vi "JKI without event handle.vi"(8 "error in":errorcluster, 10 "测试参数":string[](array[string]), 11 "测试命令":string[](array[string])) -> (0 "error out":errorcluster, 3 "执行程序":string)   [LabVIEW 2017]
doc: "函数名称： \n函数功能：无事件结构 JKI状态机模板\n入口参数：\n出口参数：\n创建时间：2018-8-17 编辑者 ：翁赟"
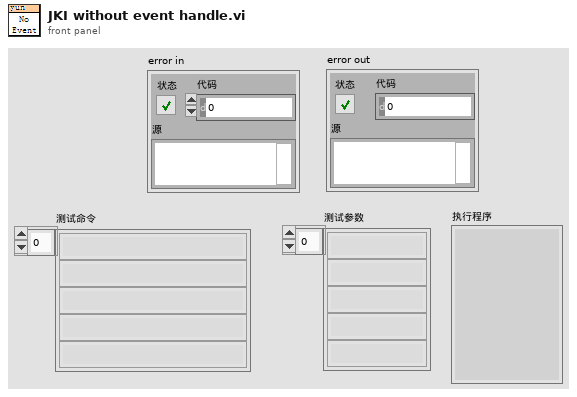
[diagram p1: front panel]
types:
  T1 = enum32{"invalid app kind", "Development System", "Run Time System", "Student Edition", "Embedded LabVIEW", "Evaluation", "Custom"}
  T2 = enum32{"Invalid", "Standard", "Closed", "Hidden", "Minimized", "Maximized"}
  T3 = cluster{"Core":cluster{"Current VI Reference":refnum<vi>, "Close Panel on Exit?":bool}, "Your Boolean data":bool, "Your string data":string}
  T4 = cluster{"Current VI Reference":refnum<vi>, "Close Panel on Exit?":bool}
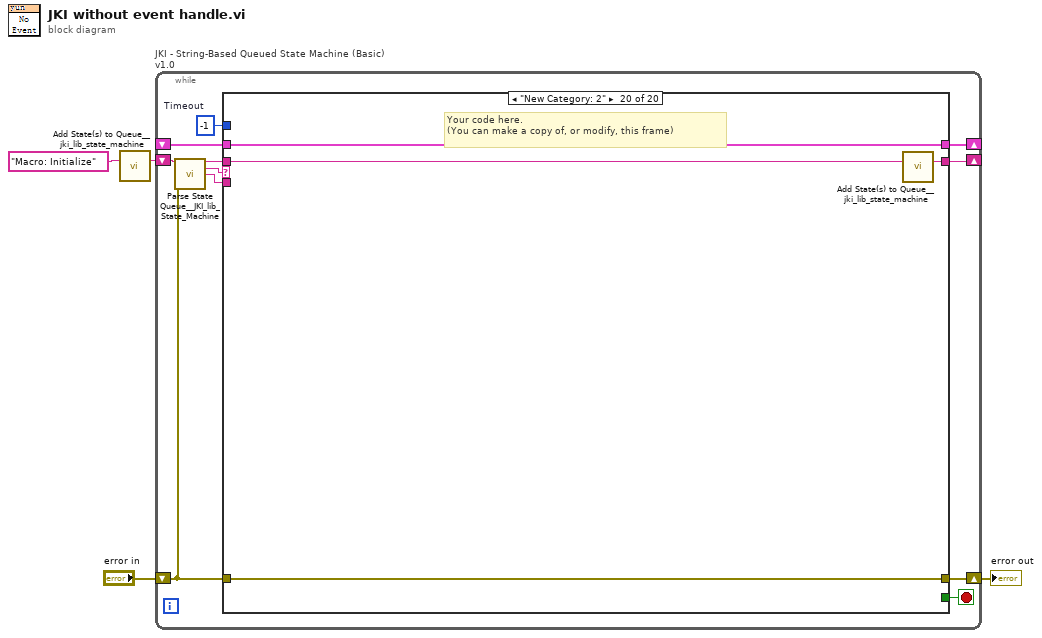
[diagram p0: block diagram]
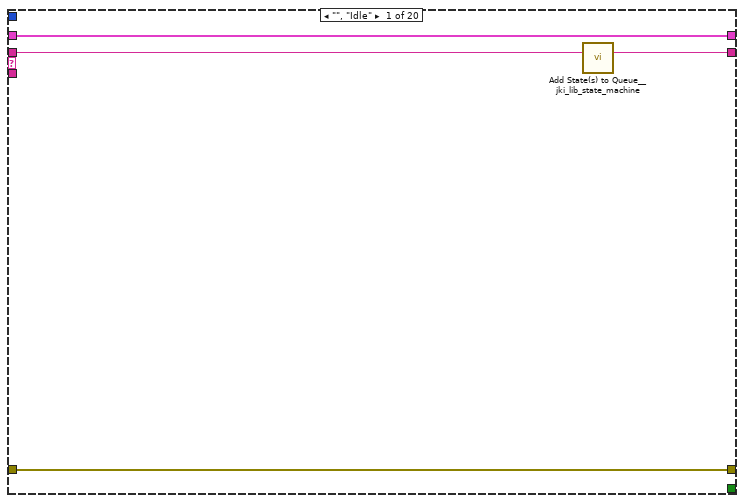
[diagram p2: hidden frame]
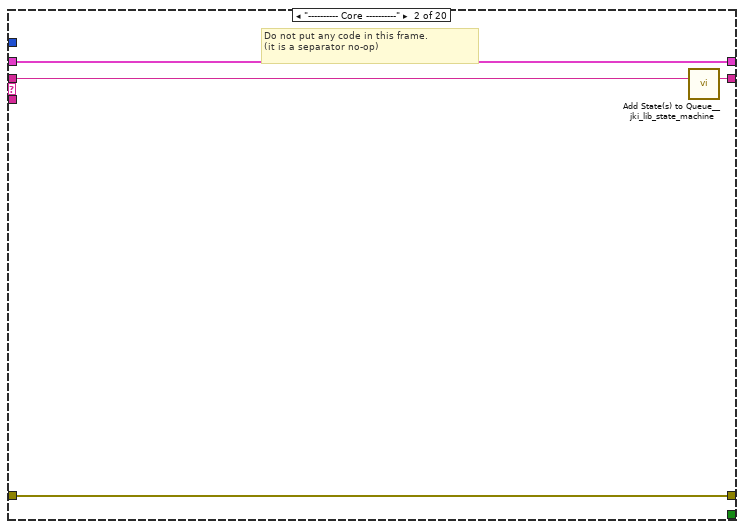
[diagram p3: hidden frame]
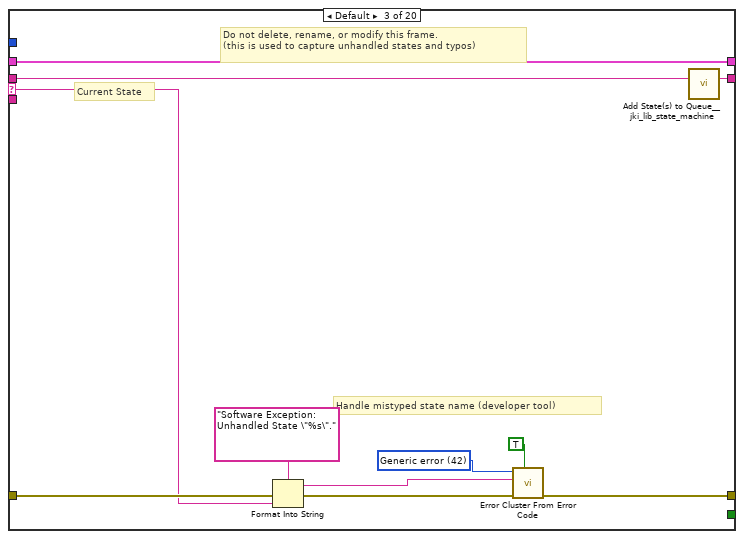
[diagram p4: hidden frame]
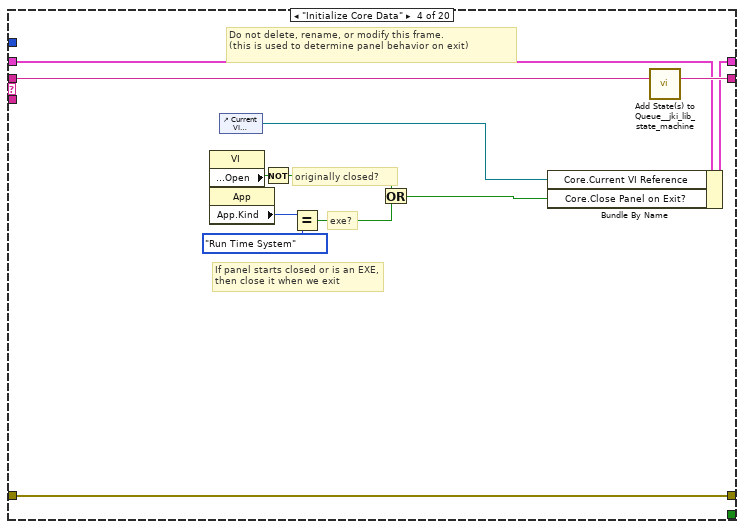
[diagram p5: hidden frame]
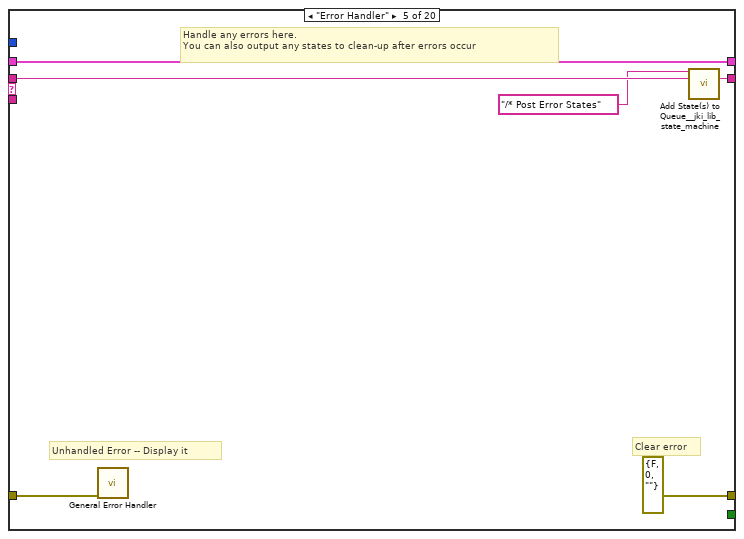
[diagram p6: hidden frame]
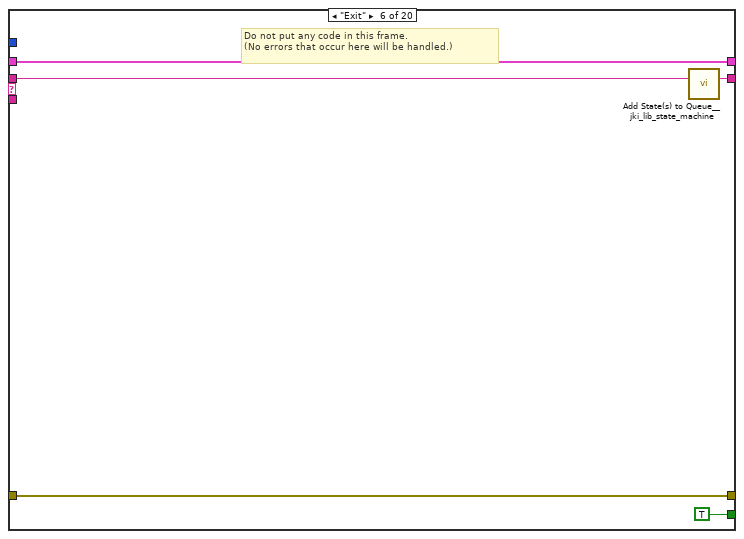
[diagram p7: hidden frame]
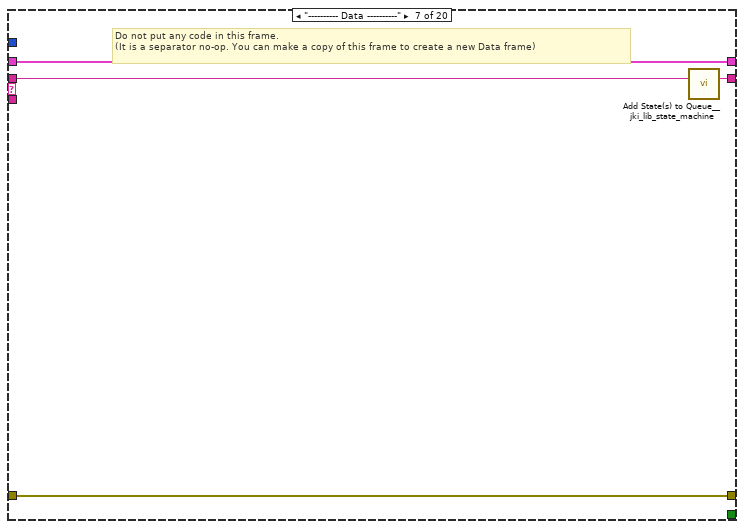
[diagram p8: hidden frame]
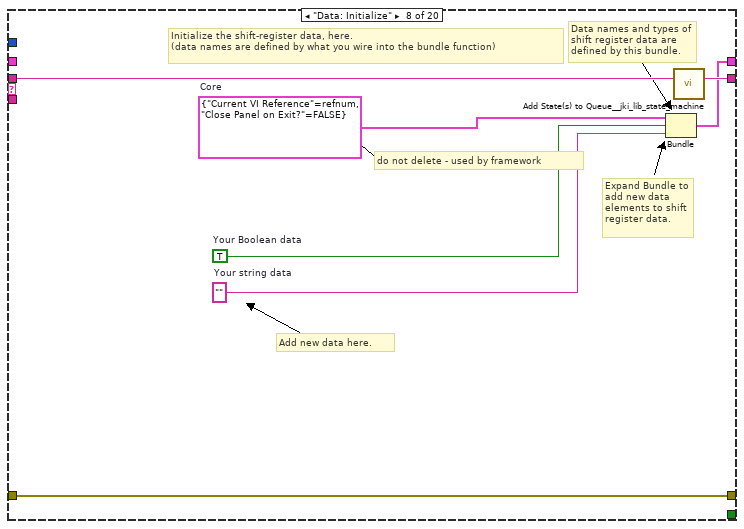
[diagram p9: hidden frame]
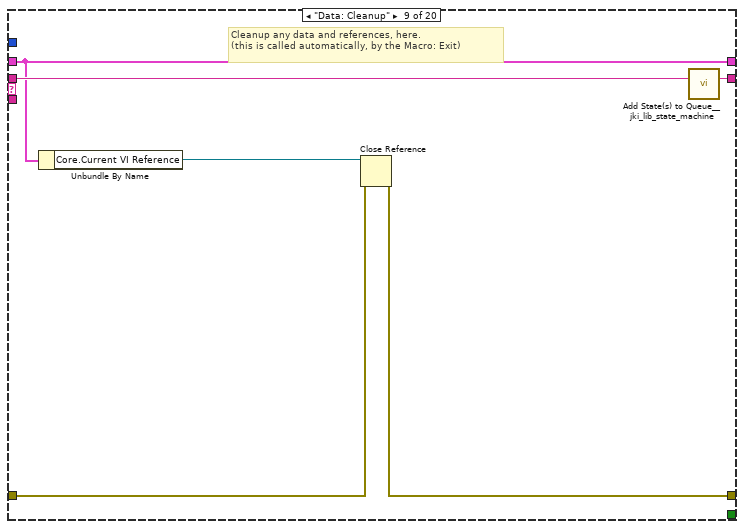
[diagram p10: hidden frame]
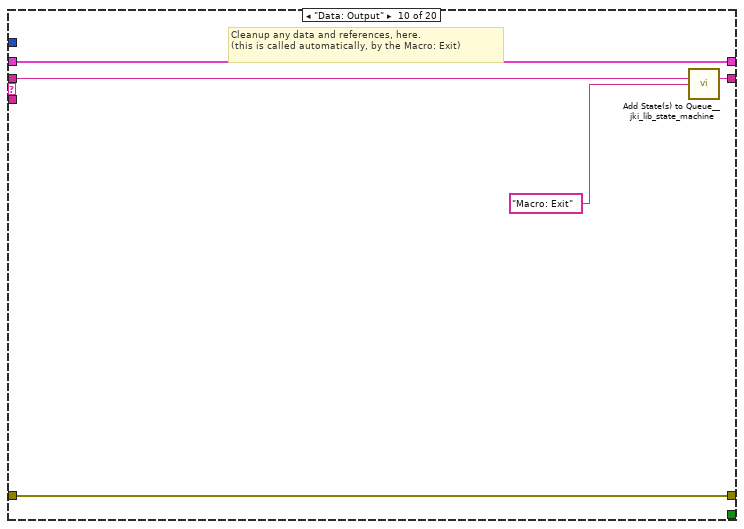
[diagram p11: hidden frame]
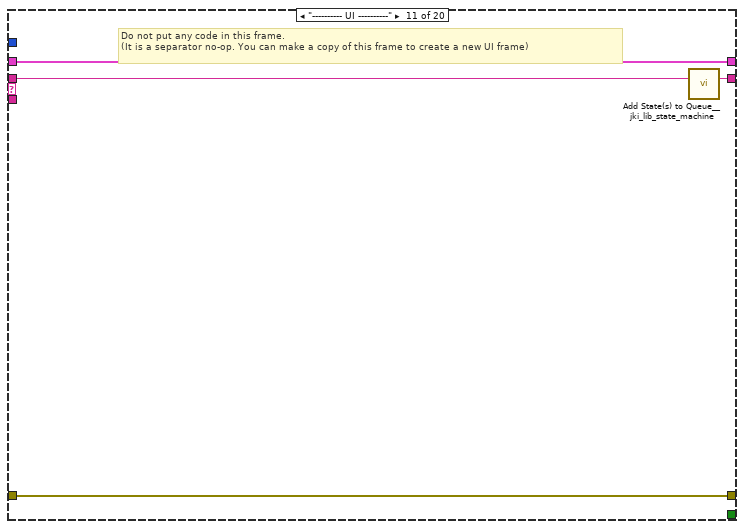
[diagram p12: hidden frame]
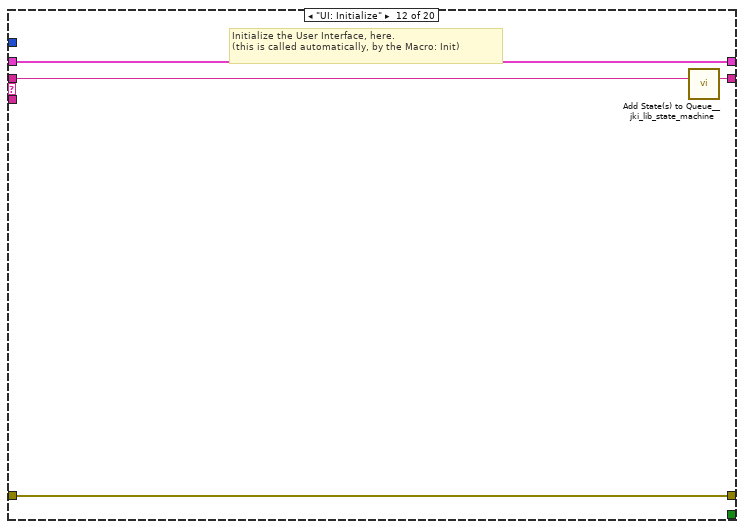
[diagram p13: hidden frame]
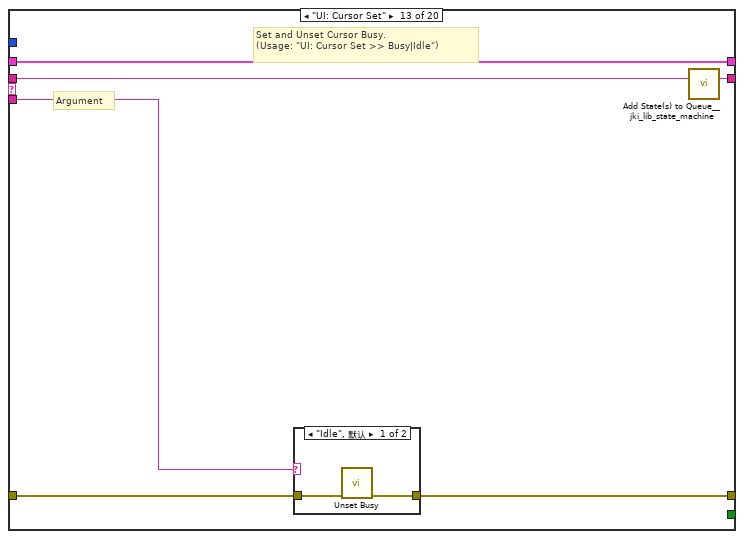
[diagram p14: hidden frame]
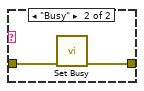
[diagram p15: hidden frame]
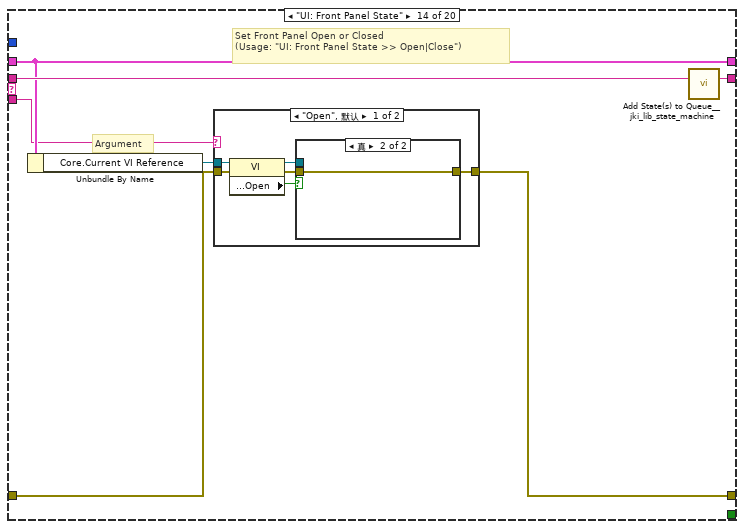
[diagram p16: hidden frame]
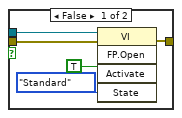
[diagram p17: hidden frame]
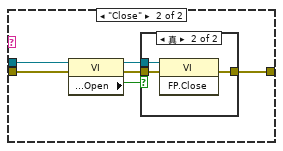
[diagram p18: hidden frame]
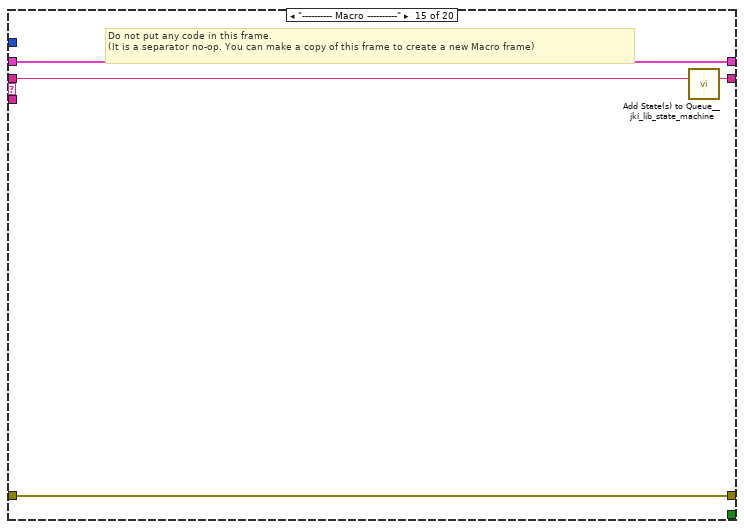
[diagram p20: hidden frame]
diagram:
  n1 = call "Add State(s) to Queue__jki_lib_state_machine.vi"("State(s) in (\"\")"="Macro: Initialize") -> ("States Out"=w4:string)  [unwired: 14 in]
  n2 = while "JKI - String-Based Queued State Machine (Basic) v1.0" {
    shift-right: [w8] -> _
    shift-left: _ -> [w7]
    shift-right: [w11] -> w1
    shift-left: "error in" -> [w5]
    shift-right: [w10] -> _
    shift-left: w4 -> [w12]
    stop <- w9 stop-if-true
    w6 = -1  # Timeout
    n3 = call "Parse State Queue__JKI_lib_State_Machine.vi"("State Queue"=w12, "Error In (no error)"=w5) -> ("Remaining States"=w14:string, "Current State"=w15:string, "Arguments"=w13:string)  [unwired: 10 in, 1 out]
    n4 = case shown="\"New Category: 2\"" w15 {
      selector: w15 -> [_ _ w24 _ _ _ _ _ _ _ _ _ _ _ _ _ _ _ _ _]
      tunnel: w14 -> [w17 w23 w28 w46 w52 w57 w61 w68 w74 w79 w83 w87 w93 w104 w130 w142 w161 w165 w169 w173]
      tunnel: w13 -> [_ _ _ _ _ _ _ _ _ _ _ _ w88 w98 _ _ _ _ _ _]
      tunnel: w7 -> [w19 w20 w26 w37 w49 w55 w58 _ w69 w77 w80 w85 w91 w100 w127 w139 w158 w162 w166 w170]
      tunnel: [w16 w21 w30 w43 errorcluster {"status"=FALSE, "code"=0, "source"=""} ("error out") w54 w59 w65 w70 w76 w81 w84 w89 w101 w128 w140 w159 w163 w167 w171] -> w11
      tunnel: w5 -> [w16 w21 w29 w43 w48 w54 w59 w65 w71 w76 w81 w84 w90 w102 w128 w140 w159 w163 w167 w171]
      tunnel: [w18 w22 w27 w45 w51 w56 w60 w67 w73 w78 w82 w86 w92 w103 w129 w141 w160 w164 w168 w172] -> w10
      tunnel: [_ _ _ _ _ TRUE _ _ _ _ _ _ _ _ _ _ _ _ _ _] -> w9
      tunnel: [w19 w20 w26 w44 w49 w55 w58 w66 w69 w77 w80 w85 w91 w100 w127 w139 w158 w162 w166 w170] -> w8
      tunnel: w6 -> [_ _ _ _ _ _ _ _ _ _ _ _ _ _ _ _ _ _ _ _]
      frame "", "Idle" {
        n5 = call "Add State(s) to Queue__jki_lib_state_machine.vi"("State(s) in (\"\")"=w17) -> ("States Out"=w18:string)  [unwired: 14 in]
      }
      frame "---------- Core ----------" {
        # "Do not put any code in this frame.\n(it is a separator no-op)"
        n6 = call "Add State(s) to Queue__jki_lib_state_machine.vi"("State(s) in (\"\")"=w23) -> ("States Out"=w22:string)  [unwired: 14 in]
      }
      frame Default {
        w33 = 42 items=["No error", "Argument error", "Memory is full", "Out of zone", "End of file", "File already open", "Generic file I/O error", "File not found", "File permission error", "Disk is full", "Duplicate path", "Too many files open", "System feature not enabled", "Resource file not found", "Cannot add resource", "Resource not found", "Image not found", "Image memory error", "Pen does not exist", "Config type invalid", "Config token not found", "Config parse error", "Config memory error", "Bad external code format", "Bad external code offset", "External code not present", "Null window", "Destroy window error", "Null menu", "Print aborted", "Bad print record", "Print driver error", "Windows error during printing", "Memory error during printing", "Print dialog error", "Generic print error", "Invalid device refnum", "Device not found", "Device parameter error", "Device unit error", "Cannot open device", "Device call aborted", "Generic error", "Cancelled by user", "Object ID too low", "Object ID too high", "Object not in heap", "Unknown heap", "Unknown object (invalid DefProc)", "Unknown object (DefProc not in table)", "Message out of range", "Invalid (null) method", "Unknown message", "Manager call not supported", "Bad address", "Network operation in progress", "Network operation timed out", "Connection is busy", "Network attribute not supported", "Network error", "Address in use", "System out of memory", "Connection aborted", "Connection refused", "Not connected", "Already connected", "Connection closed", "Initialization error (interapplication manager)", "Bad occurrence", "Wait on unbound occurrence handler", "Occurrence queue overflow", "Datalog type conflict", "Unused", "Unrecognized type (interapplication manager)", "Memory corrupt", "Failed to make temporary DLL", "Old CIN version", "Drag socket not found", "Failed to load drop-object", "Failed to register OLE object", "Failed to release OLE object", "Format specifier type mismatch", "Unknown format specifier", "Too few format specifiers", "Too many format specifiers", "Scan failed", "Newer CIN version", "Error converting to variant", "Runtime menu error", "Password tampered", "Variant attribute not found", "Incompatible variant data type", "Event data is not available", "Event Store is not present", "Occurrence is not found", "Event Queue is not created", "Event info is not available", "Refnum passed is NULL", "Error retrieving Class GUID", "Error retrieving CoClass GUID", "Error retrieving TypeLib GUID.", "Bad built application magic bytes.", "Specific driver is different from the specific driver associated with the Logical Name.", "There is no session opened to the class driver.", "Max Error", "MAX - Error with config objects", "MAX - Error loading configuration", "MAX - Group not supported"]
        # "Current State"
        # "Do not delete, rename, or modify this frame.\n(this is used to capture unhandled states and typos)"
        # "Handle mistyped state name (developer tool)"
        n7 = Format Into String(format string="Software Exception: Unhandled State \"%s\"." ("message"), error in=w29, w24) -> (resulting string=w32:string, error out=w31:errorcluster)  [unwired: 1 in]
        n8 = call <vilib>:"Error Cluster From Error Code.vi"("show call chain? (False)"=TRUE, "error in (no error)"=w31, "error message (\"\")"=w32, "error code (0)"=w33) -> ("error out"=w30:errorcluster)  [unwired: 5 in]
        n9 = call "Add State(s) to Queue__jki_lib_state_machine.vi"("State(s) in (\"\")"=w28) -> ("States Out"=w27:string)  [unwired: 14 in]
      }
      frame "Initialize Core Data" {
        # "Do not delete, rename, or modify this frame.\n(this is used to determine panel behavior on exit)"
        # "originally closed?"
        # "exe?"
        # "If panel starts closed or is an EXE, then close it when we exit"
        n10 = property class="VI"() -> ("Front Panel.Open"=w42:bool)  [unwired: 2 in, 2 out]
        n11 = property class="App"() -> ("App.Kind"=w41:T1)  [unwired: 2 in, 2 out]
        n12 = control-ref of="Current VI Reference"() -> (w35:refnum<vi>)
        n13 = Not(x=w42) -> (.not. x?=w39:bool)
        n14 = Equal?(x=w41, y=T1."Run Time System" ("Application:Kind")) -> (x = y?=w38:bool)
        n15 = Or(x=w39, y=w38) -> (x .or. y?=w36:bool)
        n16 = Bundle By Name(cluster=w37, "Core.Current VI Reference"=w35, "Core.Close Panel on Exit?"=w36) -> (w44:T3)
        n17 = call "Add State(s) to Queue__jki_lib_state_machine.vi"("State(s) in (\"\")"=w46) -> ("States Out"=w45:string)  [unwired: 14 in]
      }
      frame "Error Handler" {
        # "Unhandled Error -- Display it"
        # "Handle any errors here.\nYou can also output any states to clean-up after errors occur"
        # "Clear error"
        n18 = call <vilib>:"General Error Handler.vi"("error in (no error)"=w48) -> ()  [unwired: 10 in, 5 out]
        n19 = call "Add State(s) to Queue__jki_lib_state_machine.vi"("State(s) in Front (\"\")"="/* Post Error States", "State(s) in (\"\")"=w52) -> ("States Out"=w51:string)  [unwired: 13 in]
      }
      frame "Exit" {
        # "Do not put any code in this frame.\n(No errors that occur here will be handled.)"
        n20 = call "Add State(s) to Queue__jki_lib_state_machine.vi"("State(s) in (\"\")"=w57) -> ("States Out"=w56:string)  [unwired: 14 in]
      }
      frame "---------- Data ----------" {
        # "Do not put any code in this frame.\n(It is a separator no-op. You can make a copy of this frame to create a new Data frame)"
        n21 = call "Add State(s) to Queue__jki_lib_state_machine.vi"("State(s) in (\"\")"=w61) -> ("States Out"=w60:string)  [unwired: 14 in]
      }
      frame "Data: Initialize" {
        w62 = T4 {"Current VI Reference"=refnum, "Close Panel on Exit?"=FALSE}  # Core
        w64 = TRUE  # Your Boolean data
        w63 = ""  # Your string data
        # "do not delete - used by framework"
        # "Expand Bundle to add new data elements to shift register data."
        # "Add new data here."
        # "Data names and types of shift register data are defined by this bundle."
        # "Initialize the shift-register data, here.\n(data names are defined by what you wire into the bundle function)"
        n22 = Bundle("Core"=w62, "Your Boolean data"=w64, "Your string data"=w63) -> (w66:T3)  [unwired: 1 in]
        n23 = call "Add State(s) to Queue__jki_lib_state_machine.vi"("State(s) in (\"\")"=w68) -> ("States Out"=w67:string)  [unwired: 14 in]
      }
      frame "Data: Cleanup" {
        # "Cleanup any data and references, here.\n(this is called automatically, by the Macro: Exit)"
        n24 = Unbundle By Name(w69) -> ("Core.Current VI Reference"=w72:refnum<vi>)
        n25 = Close Reference(reference=w72, error in (no error)=w71) -> (error out=w70:errorcluster)
        n26 = call "Add State(s) to Queue__jki_lib_state_machine.vi"("State(s) in (\"\")"=w74) -> ("States Out"=w73:string)  [unwired: 14 in]
      }
      frame "Data: Output" {
        # "Cleanup any data and references, here.\n(this is called automatically, by the Macro: Exit)"
        n27 = call "Add State(s) to Queue__jki_lib_state_machine.vi"("State(s) in (\"\")"=w79, "State(s) at Back (\"\")"="Macro: Exit") -> ("States Out"=w78:string)  [unwired: 13 in]
      }
      frame "---------- UI ----------" {
        # "Do not put any code in this frame.\n(It is a separator no-op. You can make a copy of this frame to create a new UI frame)"
        n28 = call "Add State(s) to Queue__jki_lib_state_machine.vi"("State(s) in (\"\")"=w83) -> ("States Out"=w82:string)  [unwired: 14 in]
      }
      frame "UI: Initialize" {
        # "Initialize the User Interface, here.\n(this is called automatically, by the Macro: Init)"
        n29 = call "Add State(s) to Queue__jki_lib_state_machine.vi"("State(s) in (\"\")"=w87) -> ("States Out"=w86:string)  [unwired: 14 in]
      }
      frame "UI: Cursor Set" {
        # "Argument"
        # "Set and Unset Cursor Busy.\n(Usage: \"UI: Cursor Set >> Busy|Idle\")"
        n30 = case shown="\"Idle\", 默认" w88 {
          tunnel: w90 -> [w95 w97]
          tunnel: [w94 w96] -> w89
          frame "Idle", Default {
            n31 = call <vilib>:"Unset Busy.vi"("error in (no error)"=w95) -> ("error out"=w94:errorcluster)  [unwired: 10 in]
          }
          frame "Busy" {
            n32 = call <vilib>:"Set Busy.vi"("error in (no error)"=w97) -> ("error out"=w96:errorcluster)  [unwired: 9 in, 1 out]
          }
        }
        n33 = call "Add State(s) to Queue__jki_lib_state_machine.vi"("State(s) in (\"\")"=w93) -> ("States Out"=w92:string)  [unwired: 14 in]
      }
      frame "UI: Front Panel State" {
        # "Argument"
        # "Set Front Panel Open or Closed\n(Usage: \"UI: Front Panel State >> Open|Close\")"
        n34 = Unbundle By Name(w100) -> ("Core.Current VI Reference"=w99:refnum<vi>)
        n35 = case shown="\"Open\", 默认" w98 {
          tunnel: w102 -> [w108 w121]
          tunnel: [w110 w122] -> w101
          tunnel: w99 -> [w109 w119]
          frame "Open", Default {
            n36 = property class="VI"(reference=w109, error in=w108) -> (reference out=w106:refnum<vi>, error out=w107:errorcluster, "Front Panel.Open"=w105:bool)
            n37 = case shown="真" w105 {
              tunnel: [w112 w116] -> w110
              tunnel: w107 -> [w113 w116]
              tunnel: w106 -> [w111 _]
              frame False {
                n38 = invoke class="VI" method="FP.Open"(reference=w111, error in=w113, "Activate"=TRUE, "State"=T2."Standard") -> (error out=w112:errorcluster)  [unwired: 1 in, 4 out]
              }
              frame True {
              }
            }
          }
          frame "Close" {
            n39 = property class="VI"(reference=w119, error in=w121) -> (reference out=w118:refnum<vi>, error out=w120:errorcluster, "Front Panel.Open"=w117:bool)
            n40 = case shown="真" w117 {
              tunnel: [w123 w126] -> w122
              tunnel: w120 -> [w123 w125]
              tunnel: w118 -> [_ w124]
              frame False {
              }
              frame True {
                n41 = invoke class="VI" method="FP.Close"(reference=w124, error in=w125) -> (error out=w126:errorcluster)  [unwired: 1 in, 2 out]
              }
            }
          }
        }
        n42 = call "Add State(s) to Queue__jki_lib_state_machine.vi"("State(s) in (\"\")"=w104) -> ("States Out"=w103:string)  [unwired: 14 in]
      }
      frame "---------- Macro ----------" {
        # "Do not put any code in this frame.\n(It is a separator no-op. You can make a copy of this frame to create a new Macro frame)"
        n43 = call "Add State(s) to Queue__jki_lib_state_machine.vi"("State(s) in (\"\")"=w130) -> ("States Out"=w129:string)  [unwired: 14 in]
      }
      frame "Macro: Initialize" {
        w138 = "Data: Initialize\nInitialize Core Data\nUI: Initialize\n#UI: Front Panel State >> Close"  # Data: Initialize Initialize Core Data UI: Initialize #UI: Front Panel State >> Close
        n44 = Array Size(array="测试命令") -> (size(s)=w136:i32)
        n45 = for {
          N: w136 -> [_]
          tunnel: "测试命令" -> [w151]
          shift-right: [w149] -> w133
          shift-left: "" -> [w150]
          tunnel: "测试参数" -> [w148]
          i -> [w147]
          n46 = Index Array(array=w151, index=w147) -> (element=w145:string)
          n47 = Index Array(array=w148, index=w147) -> (element=w144:string)
          n48 = call "Build State String with Arguments__jki_lib_state_machine.vi"("Arguments (\"\")"=w144, "State"=w145) -> ("State with Arguments"=w143:string)  [unwired: 4 in]
          n49 = Concatenate Strings(w150, w143, "\n") -> (w149:string)
        }
        n50 = Concatenate Strings(w133, "Data: Output") -> (w131:string)
        "执行程序" <- w131
        n51 = call "Add State(s) to Queue__jki_lib_state_machine.vi"("State(s) in Front (\"\")"=w138, "State(s) in (\"\")"=w142, "State(s) at Back (\"\")"=w131) -> ("States Out"=w141:string)  [unwired: 12 in]
      }
      frame "Macro: Exit" {
        # "Exit Macro\n(This is called once, when the VI exits)"
        n52 = Unbundle By Name(w158) -> ("Core.Close Panel on Exit?"=w157:bool)
        n53 = Select(t="UI: Front Panel State >> Open", s=w157, f="") -> (s? t:f=w154:string)
        n54 = call "Add State(s) to Queue__jki_lib_state_machine.vi"("State(s) in (\"\")"=w154, "State(s) at Back (\"\")"="Data: Cleanup\nExit") -> ("States Out"=w152:string)  [unwired: 13 in]
        n55 = call "Add State(s) to Queue__jki_lib_state_machine.vi"("State(s) in Front (\"\")"=w152, "State(s) in (\"\")"=w161) -> ("States Out"=w160:string)  [unwired: 13 in]
      }
      frame "---------- New Category ----------" {
        # "Template Separator\n(You can make a copy of, or modify, this frame)"
        n56 = call "Add State(s) to Queue__jki_lib_state_machine.vi"("State(s) in (\"\")"=w165) -> ("States Out"=w164:string)  [unwired: 14 in]
      }
      frame "New Category: 1" {
        n57 = call "Add State(s) to Queue__jki_lib_state_machine.vi"("State(s) in (\"\")"=w169) -> ("States Out"=w168:string)  [unwired: 14 in]
      }
      frame "New Category: 2" {
        # "Your code here.\n(You can make a copy of, or modify, this frame)"
        n58 = call "Add State(s) to Queue__jki_lib_state_machine.vi"("State(s) in (\"\")"=w173) -> ("States Out"=w172:string)  [unwired: 14 in]
      }
    }
  }
  "error out" <- w1
